vi "BAR0469_MainProject1.vi"() -> ()   [LabVIEW 2021]
panel:
  out "Datum a cas mereni":string caption="Datum a čas měření"
  out "Actual_current":dbl caption="Aktuální proud (A)"
  out "Actual_voltage":dbl caption="Aktuální napětí (V)"
  out "V/A characteristic":cluster{dbl[], dbl[]}(graph)
  in  "Step":dbl caption="Krok (V)" min=0.0
  in  "End_voltage":dbl caption="Koncové napětí (V)" min=0.0
  in  "Intial_voltage":dbl caption="Počáteční napětí (V)" min=0.0
  in  "Start Button":bool caption="OK Button"
  in  "Stop":bool caption="OK Button"
  in  "Load":bool caption="OK Button"
  in  "Save button":bool caption="OK Button"
  in  "Reincialization Button":bool caption="OK Button"
  in  "PartType":string(combo) caption="Typ součástky"
  in  "Username":string caption="Jméno Uživatele"
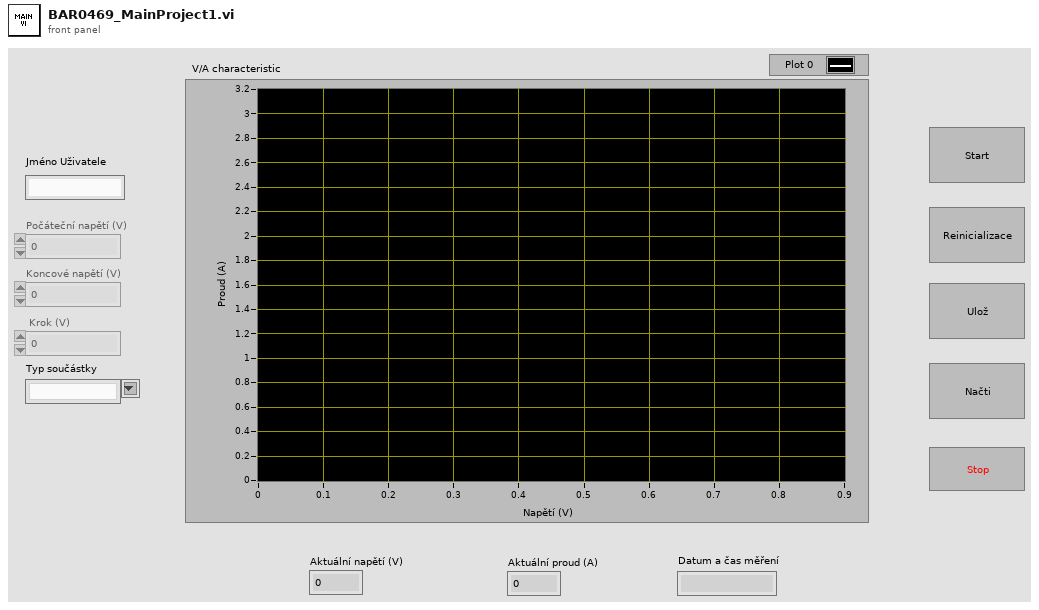
[diagram p1: front panel]
types:
  T1 = enum8{"Enabled", "Disabled", "Disabled and Grayed Out"}
  T2 = cluster{"Voltage (X)":dbl[], "Current (Y)":dbl[]}
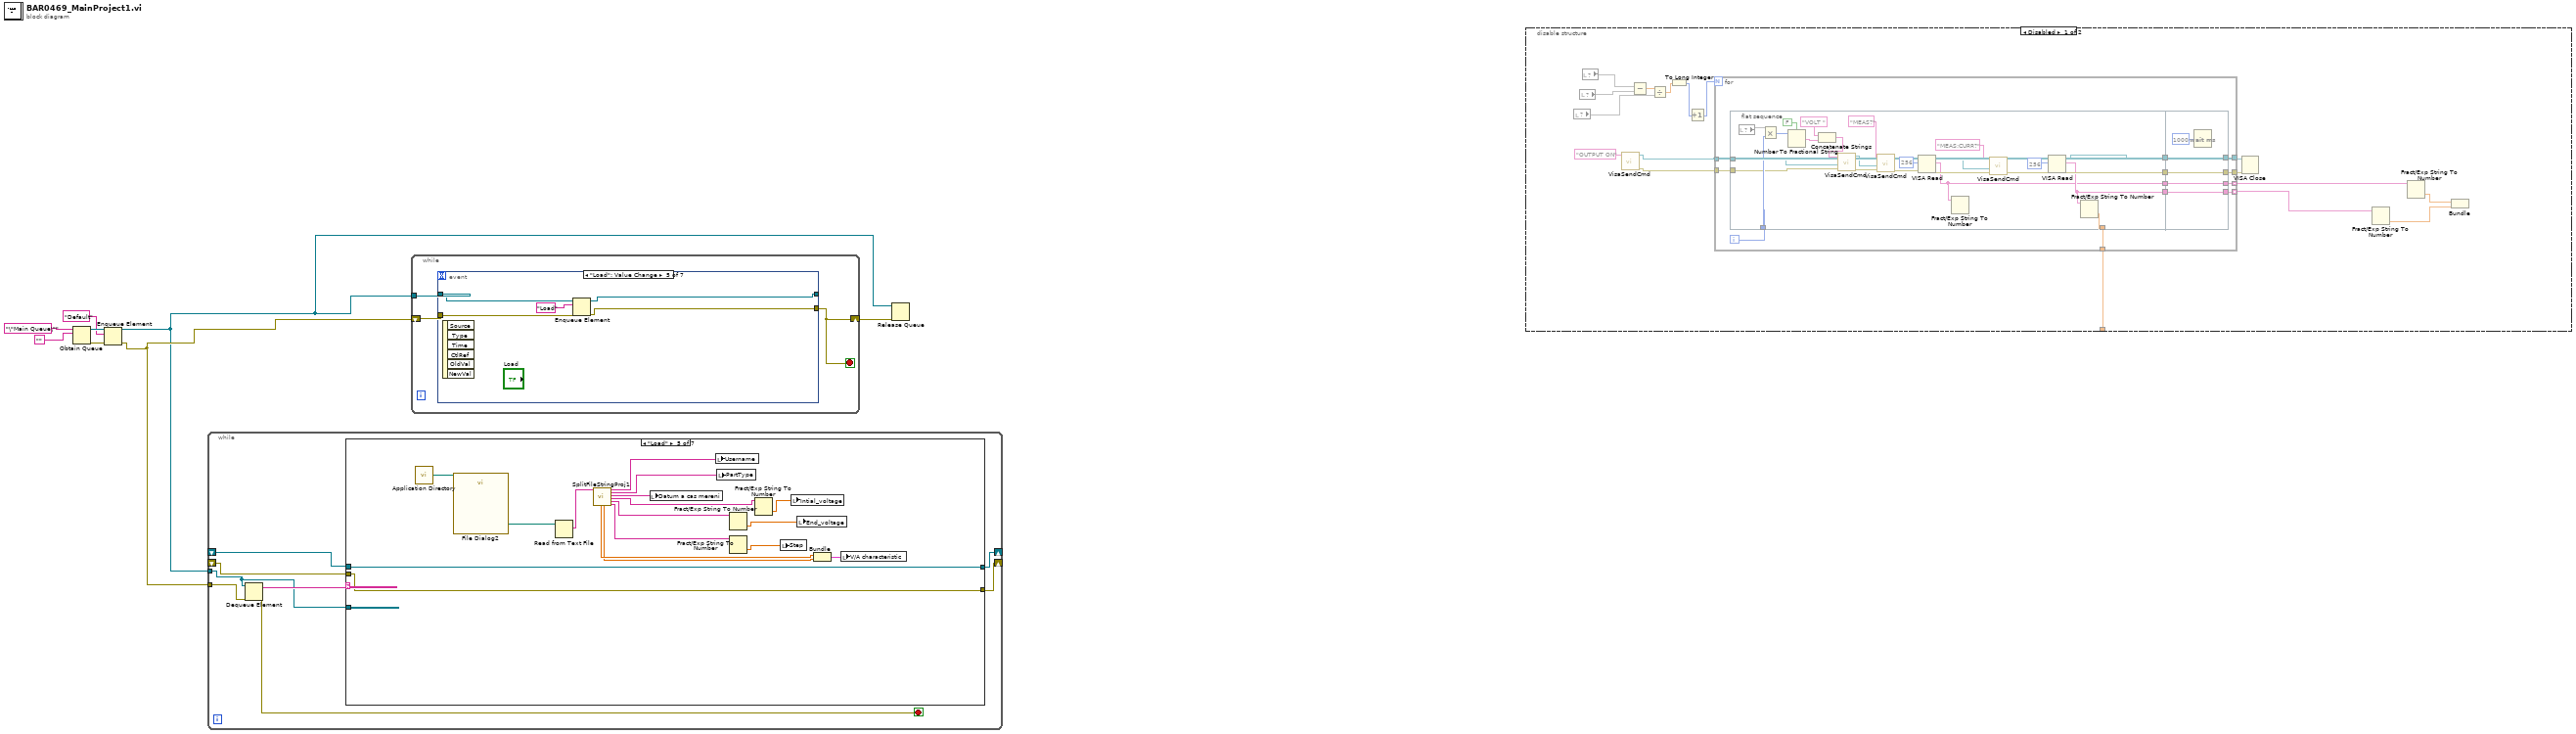
[diagram p0: block diagram]
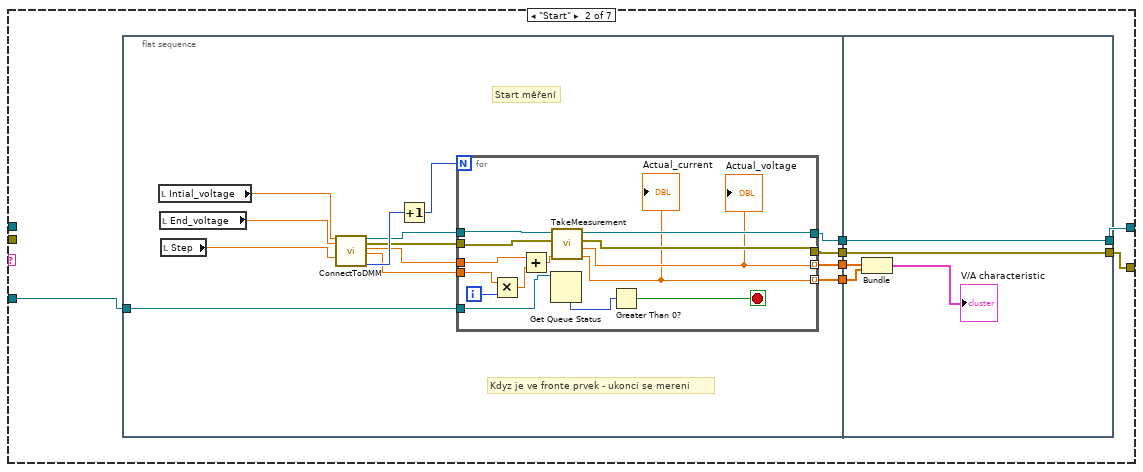
[diagram p4: hidden frame]
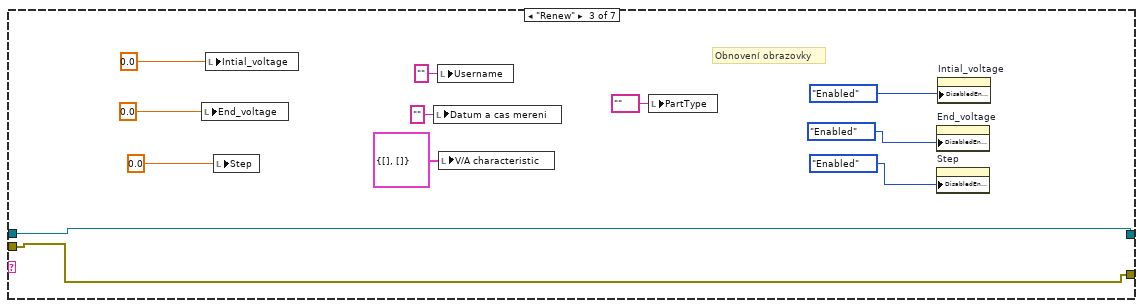
[diagram p5: hidden frame]
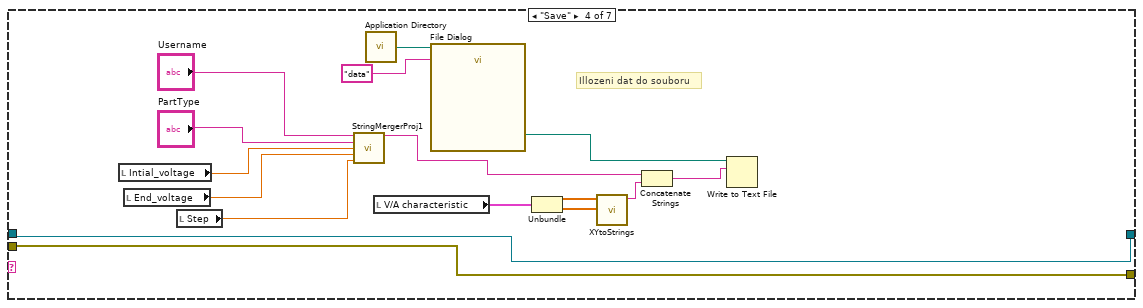
[diagram p6: hidden frame]
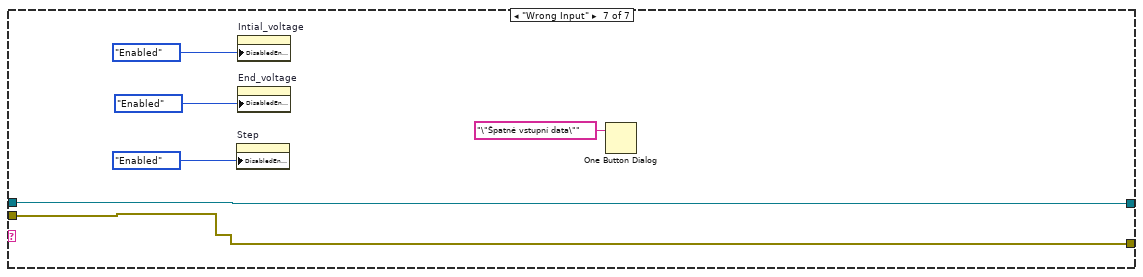
[diagram p8: hidden frame]
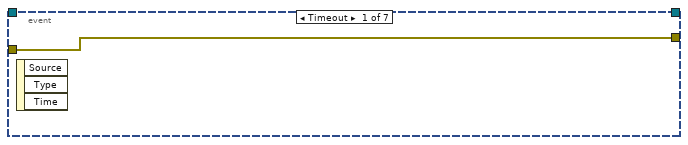
[diagram p9: hidden frame]
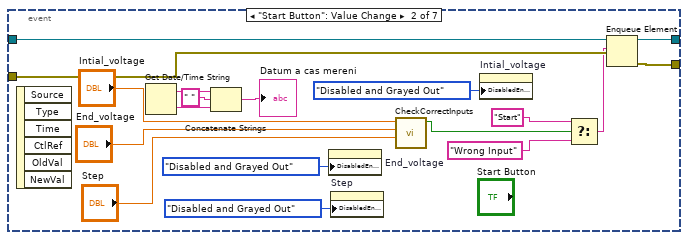
[diagram p10: hidden frame]
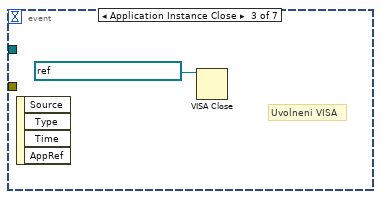
[diagram p11: hidden frame]
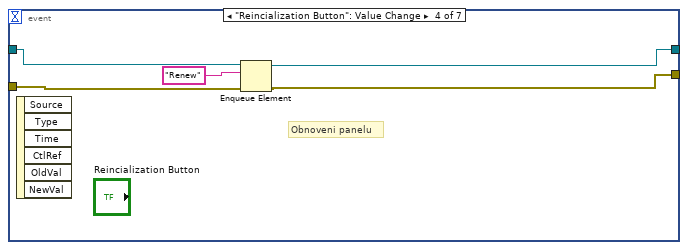
[diagram p12: hidden frame]
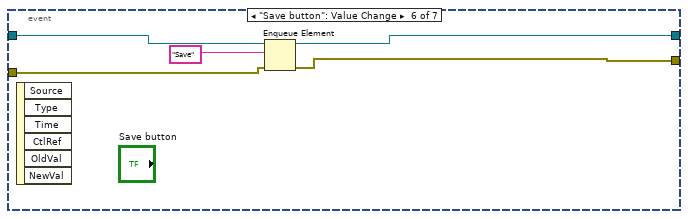
[diagram p13: hidden frame]
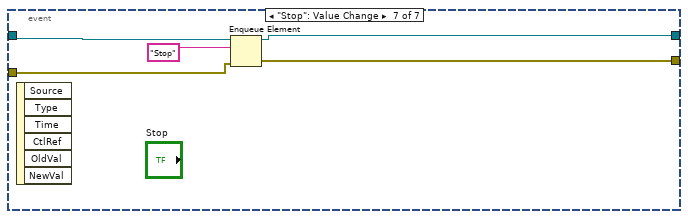
[diagram p14: hidden frame]
diagram:
  n1 = Obtain Queue(name (unnamed)="\"Main Queue\"", element data type="") -> (queue out=w6:refnum<queue>, error out=w5:errorcluster)  [unwired: 3 in, 1 out]
  n2 = Enqueue Element(queue=w6, element="Default", error in (no error)=w5) -> (queue out=w3:refnum<queue>, error out=w4:errorcluster)  [unwired: 1 in, 1 out]
  n3 = while {
    tunnel: w3 -> [w12]
    tunnel: w4 -> [w15]
    shift-right: [w11] -> _
    shift-left: _ -> [w16]
    shift-right: [w10] -> _
    shift-left: _ -> [w9]
    stop <- w14 stop-if-true
    n4 = Dequeue Element(queue=w12, error in (no error)=w15) -> (element=w13:string, error out=w14:errorcluster)  [unwired: 1 in, 2 out]
    n5 = case shown="\"Load\"" w13 {
      tunnel: [w18 w21 w67 w86 w102 w105 w111] -> w11
      tunnel: w16 -> [w18 _ w67 w86 w102 w105 w111]
      tunnel: w12 -> [_ w25 _ _ _ _ _]
      tunnel: [w17 w19 w66 w85 w101 w104 w109] -> w10
      tunnel: w9 -> [w17 _ w66 w85 w101 w104 w109]
      frame "Default", Default {
      }
      frame "Start" {
        n6 = flat-sequence {
          tunnel: w25 -> [w30]
          tunnel: [w29] -> w24
          tunnel: [w28] -> w23
          tunnel: [w27] -> w22
          tunnel: [w26] -> w20
          tunnel: w24 -> [w58]
          tunnel: w23 -> [w57]
          tunnel: [w55] -> w21
          tunnel: w22 -> [w55]
          tunnel: [w54] -> w19
          tunnel: w20 -> [w54]
          frame #0 {
            # "Kdyz je ve fronte prvek - ukonci se mereni"
            # "Start měření"
            n7 = local read "Intial_voltage"() -> (w31:dbl)
            n8 = local read "End_voltage"() -> (w39:dbl)
            n9 = local read "Step"() -> (w35:dbl)
            n10 = call "ConnectToDMM.vi"("Min Voltage (V)"=w31, "Max Voltage (V)"=w39, "Step (V)"=w35) -> ("VISA resource name out"=w37:refnum<visa-resource-name>, "error out"=w36:errorcluster, "Min Voltage (V) 2"=w33:dbl, "Step (V) 2"=w32:dbl, "unsigned 64bit integer"=w38:u64)  [unwired: 11 in, 1 out]
            n11 = Increment(x=w38) -> (x+1=w34:u64)
            n12 = for {
              N: w34 -> [_]
              tunnel: w37 -> [w53]
              tunnel: w36 -> [w52]
              tunnel: [w51] -> w27
              tunnel: [w50] -> w26
              tunnel: [w49] -> w29 mode=indexing
              tunnel: [w48] -> w28 mode=indexing
              tunnel: w33 -> [w44]
              tunnel: w32 -> [w43]
              tunnel: w30 -> [w40]
              i -> [w46]
              stop <- w42 stop-if-true
              n13 = Multiply(x=w43, y=w46) -> (x*y=w45:dbl)
              n14 = Add(x=w44, y=w45) -> (x+y=w47:dbl)
              n15 = Get Queue Status(queue=w40) -> (# elements in queue=w41:i32)  [unwired: 2 in, 7 out]
              n16 = call "TakeMeasurement.vi"("number"=w47, "error in (no error)"=w52, "VISA resource name"=w53) -> ("Actual_current"=w48:dbl, "Actual_voltage"=w49:dbl, "error out"=w50:errorcluster, "VISA resource output"=w51:refnum<visa-resource-name>)  [unwired: 5 in]
              "Actual_voltage" <- w49
              "Actual_current" <- w48
              n17 = Greater Than 0?(x=w41) -> (x > 0?=w42:bool)
            }
          }
          frame #1 {
            n18 = Bundle(w58, w57) -> (→"V/A characteristic":cluster{dbl[], dbl[]})  [unwired: 1 in]
          }
        }
      }
      frame "Renew" {
        # "Obnovení obrazovky"
        n19 = local write "End_voltage"(0.0 ("End_voltage")) -> ()
        n20 = local write "Intial_voltage"(0.0 ("Intial_voltage")) -> ()
        n21 = local write "Step"(0.0 ("Step")) -> ()
        n22 = local write "Datum a cas mereni"("" ("Datum a čas měření")) -> ()
        n23 = local write "Username"("" ("Username")) -> ()
        n24 = local write "V/A characteristic"(cluster{dbl[], dbl[]} {[], []} ("V/A characteristic")) -> ()
        n25 = local write "PartType"("" ("PartType")) -> ()
        n26 = property on="End_voltage" class="DigNum (strict)"("DisabledEnum"=T1."Enabled" ("Disabled")) -> ()  [unwired: 2 in, 2 out]
        n27 = property on="Step" class="DigNum (strict)"("DisabledEnum"=T1."Enabled" ("Disabled")) -> ()  [unwired: 2 in, 2 out]
        n28 = property on="Intial_voltage" class="DigNum (strict)"("DisabledEnum"=T1."Enabled" ("Disabled")) -> ()  [unwired: 2 in, 2 out]
      }
      frame "Save" {
        # "Illozeni dat do souboru"
        n29 = local read "Intial_voltage"() -> (w79:dbl)
        n30 = local read "End_voltage"() -> (w78:dbl)
        n31 = local read "Step"() -> (w77:dbl)
        n32 = call "StringMergerProj1.vi"("Username"="Username", "PartType"="PartType", "Min Voltage"=w79, "Max Voltage"=w78, "Step"=w77) -> ("Output string"=w71:string)  [unwired: 10 in]
        n33 = call <vilib>:"Application Directory.vi"() -> ("Application Directory"=w84:path)
        n34 = local read "V/A characteristic"() -> (w76:cluster{dbl[], dbl[]})
        n35 = call "File Dialog"("start path"=w84, "default name"="data") -> ("selected path"=w82:path)  [unwired: 10 in, 3 out]
        n36 = Unbundle(w76) -> (w75:dbl[], w74:dbl[])
        n37 = call "XYtoStrings.vi"("Array 2"=w74, "Array"=w75) -> ("concatenated string"=w72:string)  [unwired: 9 in]
        n38 = Concatenate Strings(w71, w72) -> (w73:string)
        n39 = Write to Text File(file (use dialog)=w82, text=w73) -> ()  [unwired: 2 in, 3 out]
      }
      frame "Load" {
        n40 = call <vilib>:"Application Directory.vi"() -> ("Application Directory"=w103:path)
        n41 = call "File Dialog2"("start path"=w103) -> ("selected path"=w100:path)  [unwired: 11 in, 3 out]
        n42 = Read from Text File(file (use dialog)=w100) -> (text=w99:string)  [unwired: 3 in, 3 out]
        n43 = call "SplitFileStringProj1.vi"("String from file"=w99) -> ("Voltage (X)"=w88:dbl[], "Current (Y)"=w87:dbl[], "Name"=w91:string, "Part"=w90:string, "Datum a cas mereni"=w98:string, "Minimalni napeti"=w96:string, "Maximalni napeti"=w95:string, "Krok"=w93:string)  [unwired: 11 in]
        n44 = local write "Datum a cas mereni"(w98) -> ()
        n45 = local write "Username"(w91) -> ()
        n46 = local write "PartType"(w90) -> ()
        n47 = Fract/Exp String To Number(string=w95) -> (number=w94:dbl)  [unwired: 3 in, 1 out]
        n48 = Fract/Exp String To Number(string=w93) -> (number=w92:dbl)  [unwired: 3 in, 1 out]
        n49 = Fract/Exp String To Number(string=w96) -> (number=w97:dbl)  [unwired: 3 in, 1 out]
        n50 = local write "Step"(w92) -> ()
        n51 = local write "Intial_voltage"(w97) -> ()
        n52 = local write "End_voltage"(w94) -> ()
        n53 = Bundle("Voltage (X)"=w88, "Current (Y)"=w87) -> (w89:T2)  [unwired: 1 in]
        n54 = local write "V/A characteristic"(w89) -> ()
      }
      frame "Stop" {
      }
      frame "Wrong Input" {
        n55 = property on="Step" class="DigNum (strict)"("DisabledEnum"=T1."Enabled" ("Disabled")) -> ()  [unwired: 2 in, 2 out]
        n56 = property on="Intial_voltage" class="DigNum (strict)"("DisabledEnum"=T1."Enabled" ("Disabled")) -> ()  [unwired: 2 in, 2 out]
        n57 = property on="End_voltage" class="DigNum (strict)"("DisabledEnum"=T1."Enabled" ("Disabled")) -> ()  [unwired: 2 in, 2 out]
        n58 = One Button Dialog(message="\"Špatné vstupní data\"") -> ()  [unwired: 1 in, 1 out]
      }
    }
  }
  n59 = while {
    shift-right: [w112] -> w7
    shift-left: w4 -> [w114]
    tunnel: w3 -> [w113]
    stop <- w112 stop-if-true
    n60 = event shown="[4] \"Load\": Value Change" {
      selector: _ -> [_ _ _ _ _ _ _]
      dyn-events: _ -> [_ _ _ _ _ _ _]
      timeout: _ -> [_ _ _ _ _ _ _]
      tunnel: w114 -> [w115 w133 _ w138 w141 w149 w154]
      tunnel: [w115 w132 _ w136 w142 w146 w151] -> w112
      tunnel: w113 -> [_ w131 _ w139 w144 w148 w153]
      tunnel: [_ w130 _ w137 w143 w147 w152] -> _
      event Timeout {
        n61 = event-data() -> ()  [unwired: 1 in, 3 out]
      }
      event "Start Button": Value Change {
        n62 = event-data() -> ()  [unwired: 1 in, 6 out]
        n63 = Get Date/Time String() -> (date string=w119:string, time string=w116:string)  [unwired: 3 in]
        n64 = Concatenate Strings(w119, " " ("string"), w116) -> (→"Datum a cas mereni":string)
        n65 = property on="End_voltage" class="DigNum (strict)"("DisabledEnum"=T1."Disabled and Grayed Out" ("Disabled")) -> ()  [unwired: 2 in, 2 out]
        n66 = property on="Step" class="DigNum (strict)"("DisabledEnum"=T1."Disabled and Grayed Out" ("Disabled")) -> ()  [unwired: 2 in, 2 out]
        n67 = call "CheckCorrectInputs.vi"("Step"="Step", "Max"="End_voltage", "Min"="Intial_voltage") -> ("x .or. y?"=w127:bool)  [unwired: 8 in]
        n68 = property on="Intial_voltage" class="DigNum (strict)"("DisabledEnum"=T1."Disabled and Grayed Out" ("Disabled")) -> ()  [unwired: 2 in, 2 out]
        n69 = Select(t="Start", s=w127, f="Wrong Input") -> (s? t:f=w126:string)
        n70 = Enqueue Element(queue=w131, element=w126, error in (no error)=w133) -> (queue out=w130:refnum<queue>, error out=w132:errorcluster)  [unwired: 1 in, 1 out]
      }
      event Application Instance Close {
        # "Uvolneni VISA"
        n71 = event-data() -> ()  [unwired: 1 in, 4 out]
        n72 = VISA Close(VISA resource name=refnum<visa-resource-name> "DMMandPowerSupply") -> ()  [unwired: 1 in, 1 out]
      }
      event "Reincialization Button": Value Change {
        # "Obnoveni panelu"
        n73 = event-data() -> ()  [unwired: 1 in, 6 out]
        n74 = Enqueue Element(queue=w139, element="Renew", error in (no error)=w138) -> (queue out=w137:refnum<queue>, error out=w136:errorcluster)  [unwired: 1 in, 1 out]
      }
      event "Load": Value Change {
        n75 = event-data() -> ()  [unwired: 1 in, 6 out]
        n76 = Enqueue Element(queue=w144, element="Load", error in (no error)=w141) -> (queue out=w143:refnum<queue>, error out=w142:errorcluster)  [unwired: 1 in, 1 out]
      }
      event "Save button": Value Change {
        n77 = event-data() -> ()  [unwired: 1 in, 6 out]
        n78 = Enqueue Element(queue=w148, element="Save", error in (no error)=w149) -> (queue out=w147:refnum<queue>, error out=w146:errorcluster)  [unwired: 1 in, 1 out]
      }
      event "Stop": Value Change {
        n79 = event-data() -> ()  [unwired: 1 in, 6 out]
        n80 = Enqueue Element(queue=w153, element="Stop", error in (no error)=w154) -> (queue out=w152:refnum<queue>, error out=w151:errorcluster)  [unwired: 1 in, 1 out]
      }
    }
  }
  n81 = Release Queue(queue=w3, error in (no error)=w7) -> ()  [unwired: 1 in, 3 out]
  n82 = disable-structure shown="Disabled" {
    disable-tunnel: [w155 _] -> _
    frame Disabled {
      n83 = local read item#-1() -> (w168)
      n84 = local read item#-1() -> (w170)
      n85 = local read item#-1() -> (w171)
      n86 = call "VisaSendCmd.vi"("Msg to send"="OUTPUT ON") -> ("error out"=w160:errorcluster, "VISA resource output"=w161:refnum<visa-resource-name>)  [unwired: 9 in]
      n87 = Subtract(x=w171, y=w170) -> (x-y=w169:dbl)
      n88 = Divide(x=w169, y=w168) -> (x/y=w167:dbl)
      n89 = To Long Integer(number=w167) -> (32bit integer=w165:i32)
      n90 = Increment(x=w165) -> (x+1=w166:i32)
      n91 = for {
        N: w166 -> [_]
        tunnel: [w181] -> w163
        tunnel: [w180] -> w162
        tunnel: w161 -> [w178]
        tunnel: w160 -> [w177]
        tunnel: [w175] -> w156 mode=indexing
        tunnel: [w173] -> w157 mode=indexing
        tunnel: [w172] -> w155
        i -> [w183]
        n92 = flat-sequence {
          tunnel: w183 -> [w205]
          tunnel: [w193] -> w182
          tunnel: [w192] -> w179
          tunnel: w178 -> [w189]
          tunnel: w177 -> [w188]
          tunnel: [w186] -> w176
          tunnel: [w187] -> w174
          tunnel: [w184] -> w172
          tunnel: w182 -> [w214]
          tunnel: [w214] -> w181
          tunnel: [w213] -> w180
          tunnel: w179 -> [w213]
          tunnel: [w211] -> w175
          tunnel: w176 -> [w211]
          tunnel: w174 -> [w210]
          tunnel: [w210] -> w173
          frame #0 {
            n93 = local read item#-1() -> (w204)
            n94 = Multiply(x=w204, y=w205) -> (x*y=w206:i32)
            n95 = Number To Fractional String(use system decimal point (T)=FALSE, number=w206) -> (F-format string=w207:string)  [unwired: 2 in]
            n96 = Concatenate Strings("VOLT ", w207) -> (w209:string)
            n97 = call "VisaSendCmd.vi"("error in (no error)"=w188, "VISA resource name"=w189, "Msg to send"=w209) -> ("error out"=w202:errorcluster, "VISA resource output"=w203:refnum<visa-resource-name>)  [unwired: 7 in]
            n98 = call "VisaSendCmd.vi"("error in (no error)"=w202, "VISA resource name"=w203, "Msg to send"="MEAS?") -> ("error out"=w200:errorcluster, "VISA resource output"=w201:refnum<visa-resource-name>)  [unwired: 7 in]
            n99 = VISA Read(VISA resource name=w201, byte count=u32 256, error in (no error)=w200) -> (VISA resource name out=w191:refnum<visa-resource-name>, read buffer=w186:string, error out=w190:errorcluster)  [unwired: 1 out]
            n100 = Fract/Exp String To Number(string=w186) -> ()  [unwired: 3 in, 2 out]
            n101 = call "VisaSendCmd.vi"("error in (no error)"=w190, "VISA resource name"=w191, "Msg to send"="MEAS:CURR?") -> ("error out"=w195:errorcluster, "VISA resource output"=w196:refnum<visa-resource-name>)  [unwired: 7 in]
            n102 = VISA Read(VISA resource name=w196, byte count=u32 256, error in (no error)=w195) -> (VISA resource name out=w193:refnum<visa-resource-name>, read buffer=w187:string, error out=w192:errorcluster)  [unwired: 1 out]
            n103 = Fract/Exp String To Number(string=w187) -> (number=w184:dbl)  [unwired: 3 in, 1 out]
          }
          frame #1 {
            n104 = Wait (ms)(milliseconds to wait=u32 1000) -> ()  [unwired: 1 out]
          }
        }
      }
      n105 = VISA Close(VISA resource name=w163, error in (no error)=w162) -> ()  [unwired: 1 out]
      n106 = Fract/Exp String To Number(string=w157) -> (number=w158:dbl[])  [unwired: 3 in, 1 out]
      n107 = Fract/Exp String To Number(string=w156) -> (number=w159:dbl[])  [unwired: 3 in, 1 out]
      n108 = Bundle(w159, w158) -> ()  [unwired: 1 in, 1 out]
    }
    frame Enabled {
    }
  }
